vi "Writing direction.vi"(0 "PDF Report IN":refnum<class "PDF Report Class.lvclass">, 2 "Text type":T1, 5 "Phrase refnum":refnum<k24>, 7 "Paragraph refnum":refnum<k24>, 9 "ChapterAutoNumber":refnum<k24>, 11 "error in (no error)":errorcluster, 12 "Section":refnum<k24>, 13 "Title":string) -> (4 "PDF Report OUT":refnum<class "PDF Report Class.lvclass">, 15 "error out":errorcluster)   [LabVIEW 2020, in "Exaprom PDF.lvlib"]
doc: "Version 2.0\nDeveloped by Jean-Marc Simard\nCopyright © 2013, Exaprom Inc.\nAll rights reserved.\nLicense: BSD\n\nWith iTextSharp 4.1.6 (http://itextsharp.sourceforge.net)\nunder Mozilla Public License Version 1.1\n(http://www.mozilla.org/MPL/MPL-1.1.html)"
uses:
  <userlib>/labview-PDF-writer-master/Exaprom PDF.lvlib
  <userlib>/labview-PDF-writer-master/LV Class/PDF Report Class/PDF Report Class.lvclass
  C:/Program Files (x86)/National Instruments/LabVIEW 2020/user.lib/labview-PDF-writer-master/DLL/itextsharp.dll
  DLL/itextsharp.dll
  <userlib>/labview-PDF-writer-master/Controls/Text Controls/Unicode/Type and run direction.ctl
  <userlib>/labview-PDF-writer-master/LV Class/Fonts Class/Font Class.lvclass
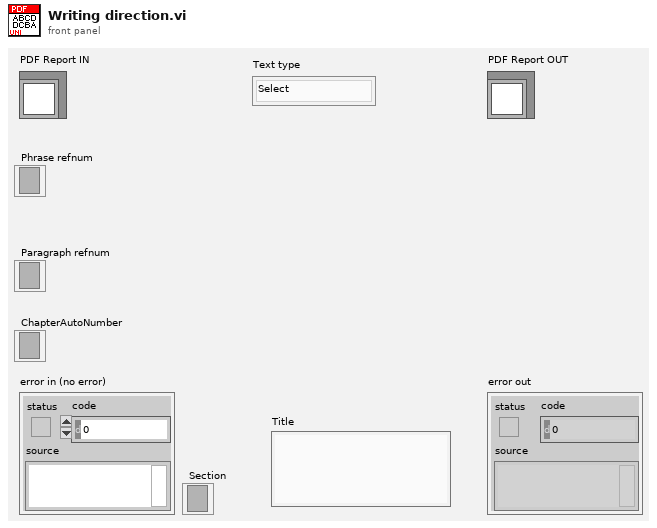
[diagram p1: front panel]
types:
  T1 = typedef "Exaprom PDF.lvlib/Type and run direction.ctl" = enum16{"Select", "ASCII", "UTF-16", "UTF-16 (default)", "UTF-16 (LTR)", "UTF-16 (RTL)"}
  T2 = typedef "Exaprom PDF.lvlib/Font complete cluster.ctl" = cluster{"Name":string, "Size":T3, "Color":T4, "Style":cluster{"Bold":bool, "Italic":bool, "Underline":bool, "Strikeout":bool}, "Type":T5}
  T3 = typedef "Exaprom PDF.lvlib/Font size.ctl" = sgl
  T4 = typedef "Exaprom PDF.lvlib/Font color.ctl" = u32
  T5 = typedef "Exaprom PDF.lvlib/Type and encoding.ctl" = cluster{"Type&direction":T1, "Embedded":bool, "Encoding":string}
  T6 = typedef "Exaprom PDF.lvlib/Page dimensions.ctl" = cluster{"Start at page":i32, "Page Size":T7, "Orientation":T8, "widht":sgl, "height":sgl, "Margin left":sgl, "Margin right":sgl, "Margin top":sgl, "Margin bottom":sgl, "X0":sgl, "X1":sgl, "Y0":sgl, "Y1":sgl}
  T7 = typedef "Exaprom PDF.lvlib/Page size.ctl" = i32
  T8 = typedef "Exaprom PDF.lvlib/Page Orientation.ctl" = enum16{"Portrait", "Landscape"}
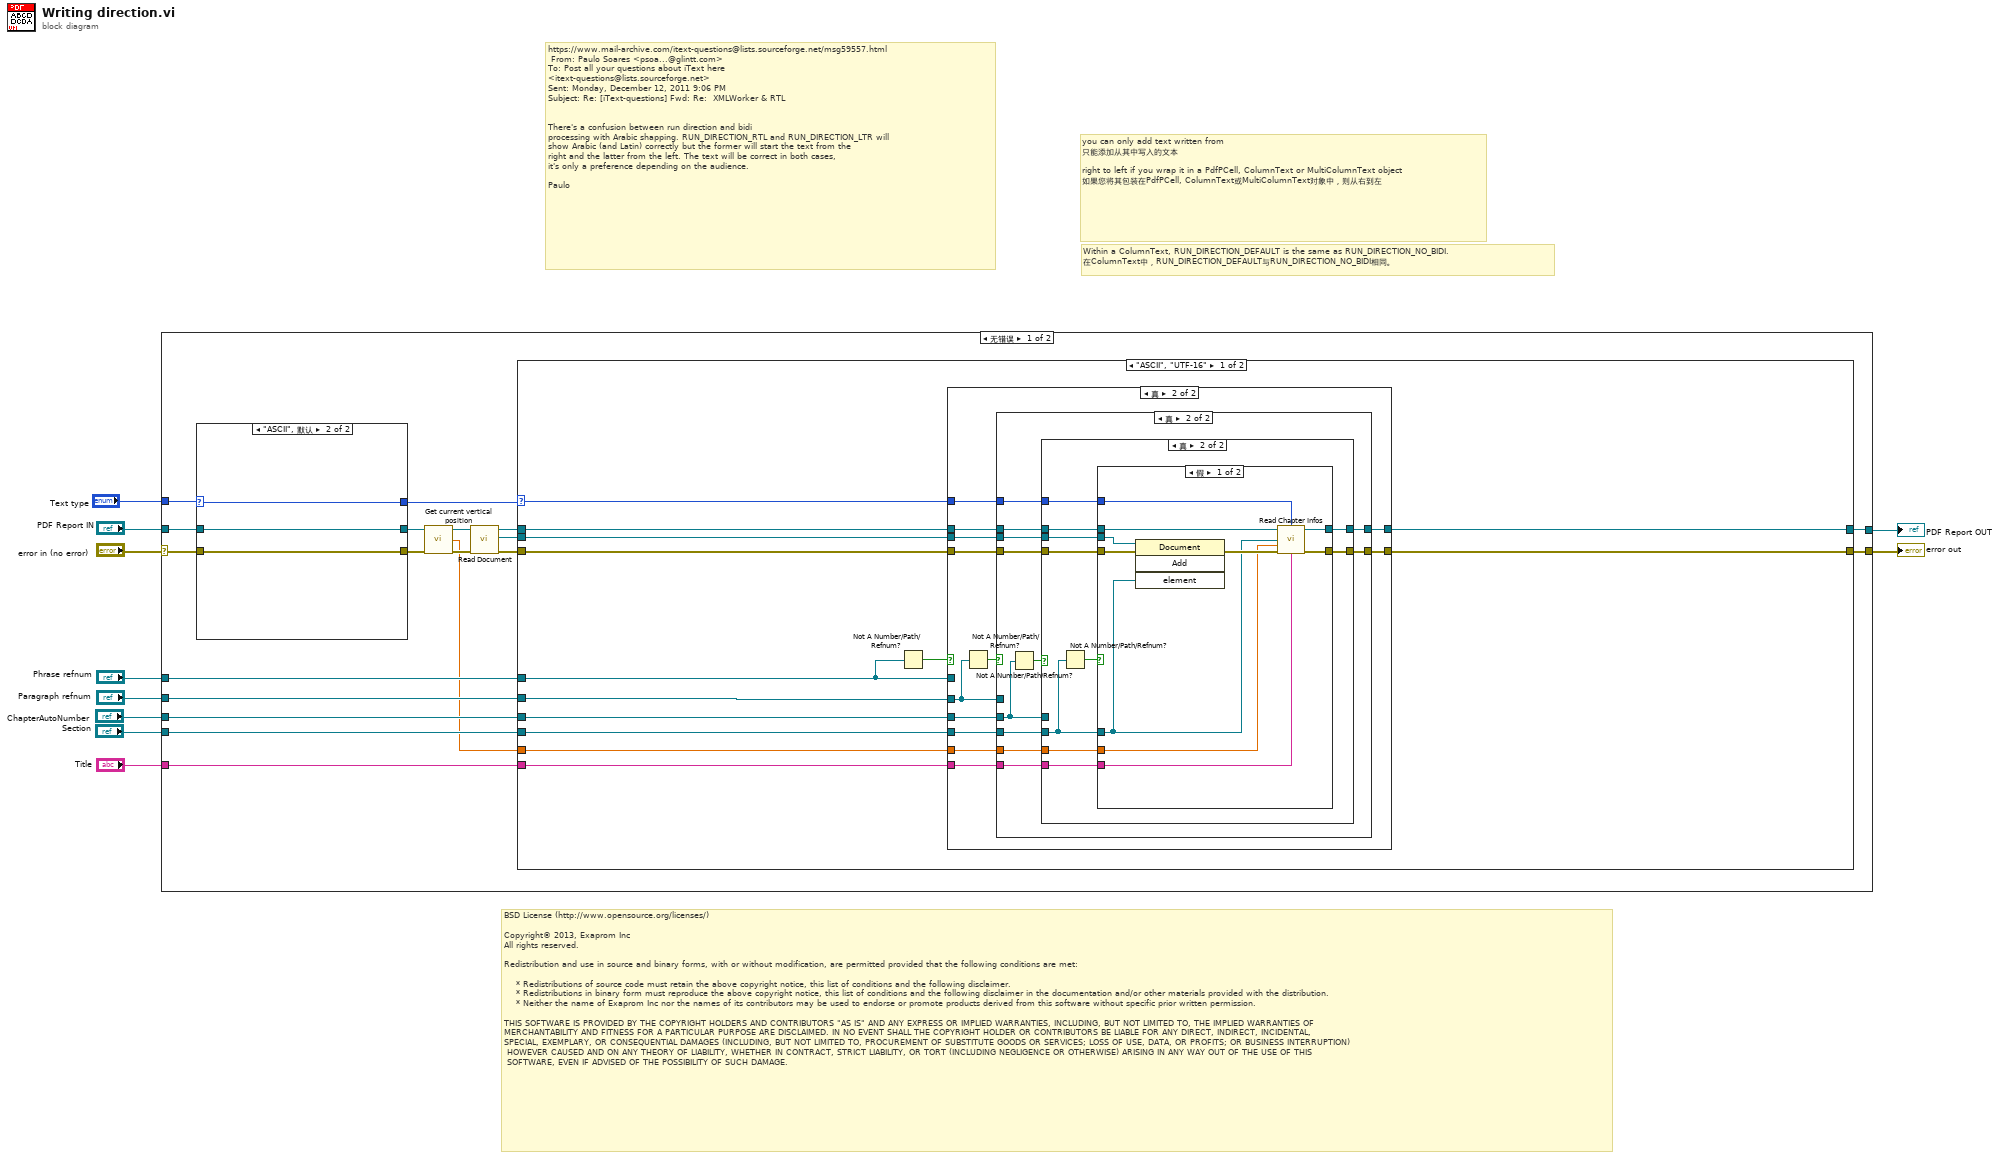
[diagram p0: block diagram]
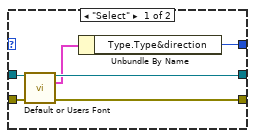
[diagram p2: hidden frame]
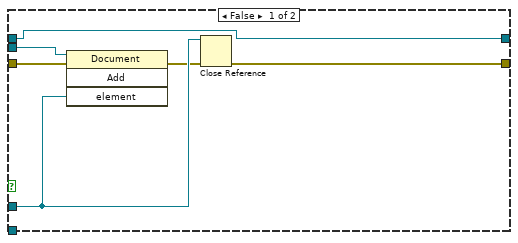
[diagram p3: hidden frame]
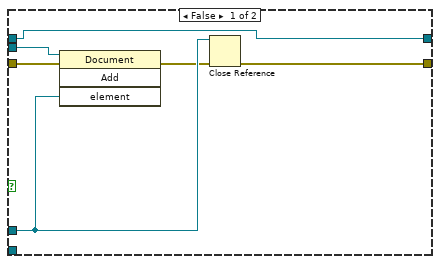
[diagram p4: hidden frame]
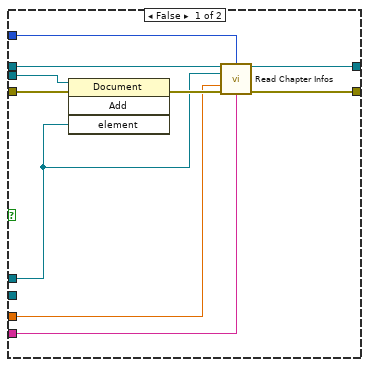
[diagram p5: hidden frame]
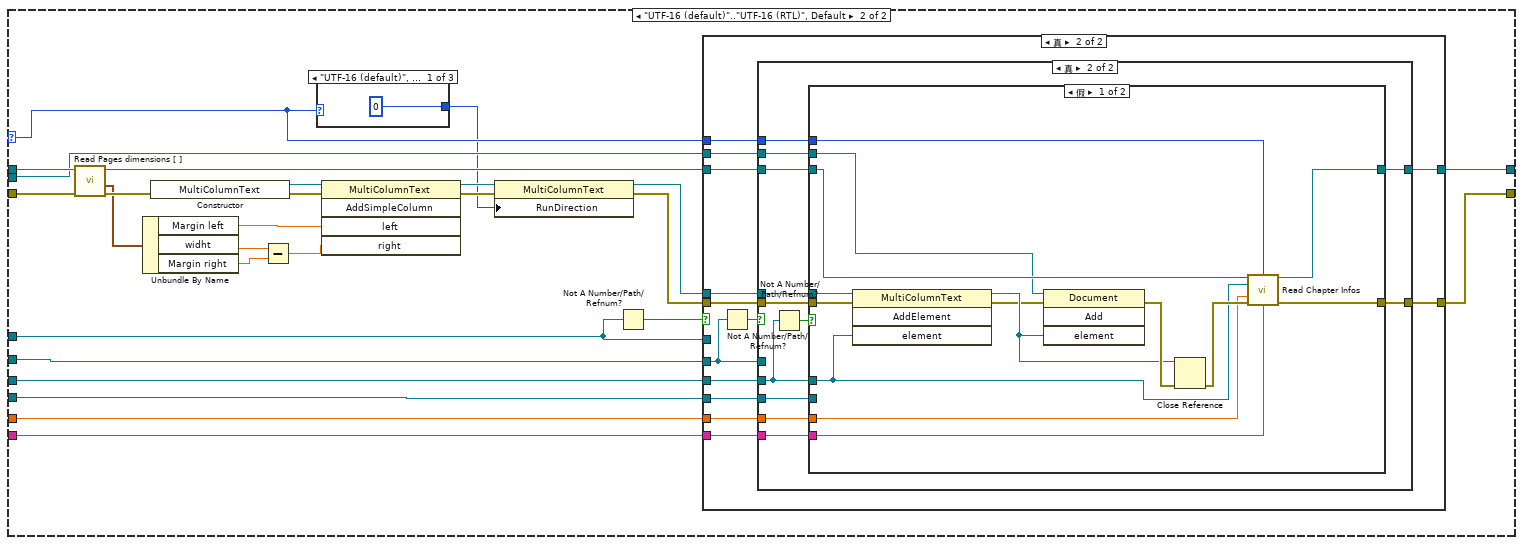
[diagram p7: hidden frame]
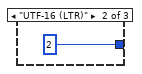
[diagram p8: hidden frame]
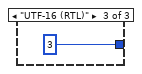
[diagram p9: hidden frame]
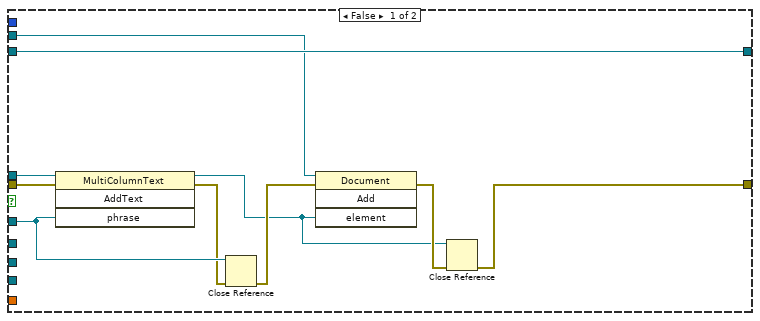
[diagram p10: hidden frame]
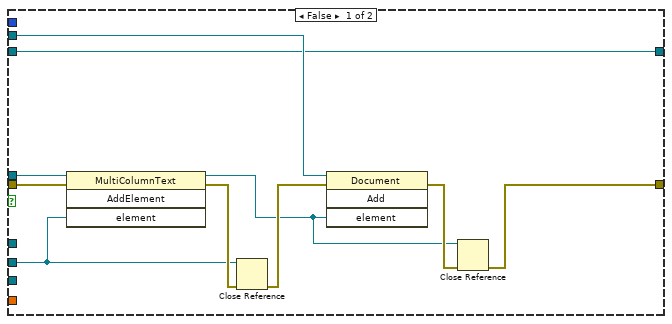
[diagram p11: hidden frame]
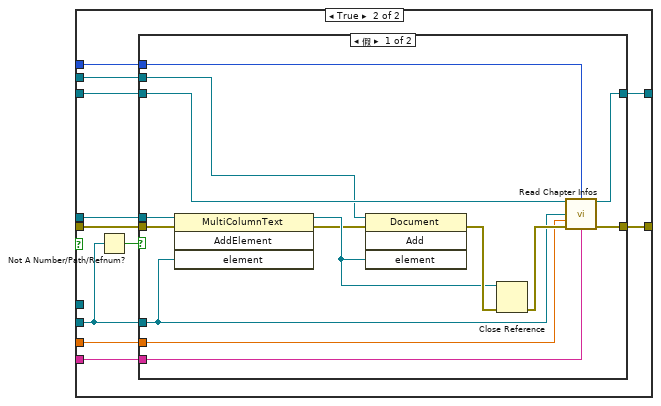
[diagram p12: hidden frame]
diagram:
  # "Within a ColumnText, RUN_DIRECTION_DEFAULT is the same as RUN_DIRECTION_NO_BIDI.\n在ColumnText中，RUN_DIRECTION_DEFAULT与RUN_DIRECTION_NO_BIDI相同。"
  # "you can only add text written from \n只能添加从其中写入的文本\n\nright to left if you wrap it in a PdfPCell, ColumnText or MultiColumnText object\n如果您将其包装在PdfPCell, ColumnText或MultiColumnText对象中，则从右到左"
  # "https://www.mail-archive.com/itext-questions@lists.sourceforge.net/msg59557.html\n From: Paulo Soares <psoa...@glintt.com>\nTo: Post all your questions about iText here \n<itext-questions@lists.sourceforge.net> \nSent: Monday, December 12, 2011 9:06 PM\nSubject: Re: [iText-questions] Fwd: Re:  XMLWorker & RTL\n \n\nThere's a confusion between run direction and bidi \nprocessing with Arabic shapping. RUN_DIRECTION_RTL and RUN_DIRECTION_LTR will \nshow Arabic (and Latin) correctly but the former will start the text from the \nright and the latter from the left. The text will be correct in both cases, \nit's only a preference depending on the audience.\n \nPaulo"
  # "BSD License (http://www.opensource.org/licenses/)\n\nCopyright© 2013, Exaprom Inc\nAll rights reserved.\n\nRedistribution and use in source and binary forms, with or without modification, are permitted provided that the following conditions are met:\n\n    * Redistributions of source code must retain the above copyright notice, this list of conditions and the following disclaimer.\n    * Redistributions in binary form must reproduce the above copyright notice, this list of conditions and the following disclaimer in the documentation and/or other materials provided with the distribution.\n    * Neither the name of Exaprom Inc nor the names of its contributors may be used to endorse or promote products derived from this software without specific prior written permission.\n\nTHIS SOFTWARE IS PROVIDED BY THE COPYRIGHT HOLDERS AND CONTRIBUTORS \"AS IS\" AND ANY EXPRESS OR IMPLIED WARRANTIES, INCLUDING, BUT NOT LIMITED TO, THE IMPLIED WARRANTIES OF \nMERCHANTABILITY AND FITNESS FOR A PARTICULAR PURPOSE ARE DISCLAIMED. IN NO EVENT SHALL THE COPYRIGHT HOLDER OR CONTRIBUTORS BE LIABLE FOR ANY DIRECT, INDIRECT, INCIDENTAL,\nSPECIAL, EXEMPLARY, OR CONSEQUENTIAL DAMAGES (INCLUDING, BUT NOT LIMITED TO, PROCUREMENT OF SUBSTITUTE GOODS OR SERVICES; LOSS OF USE, DATA, OR PROFITS; OR BUSINESS INTERRUPTION)\n HOWEVER CAUSED AND ON ANY THEORY OF LIABILITY, WHETHER IN CONTRACT, STRICT LIABILITY, OR TORT (INCLUDING NEGLIGENCE OR OTHERWISE) ARISING IN ANY WAY OUT OF THE USE OF THIS\n SOFTWARE, EVEN IF ADVISED OF THE POSSIBILITY OF SUCH DAMAGE."
  n1 = case shown="无错误" "error in (no error)" {
    selector: "error in (no error)" -> [w13 w236]
    tunnel: "PDF Report IN" -> [w14 w235]
    tunnel: [w28 w235] -> w9
    tunnel: [w29 w236] -> w8
    tunnel: "Phrase refnum" -> [w27 _]
    tunnel: "Paragraph refnum" -> [w26 _]
    tunnel: "Text type" -> [w16 _]
    tunnel: "ChapterAutoNumber" -> [w22 _]
    tunnel: "Section" -> [w21 _]
    tunnel: "Title" -> [w17 _]
    frame No Error {
      n2 = case shown="\"ASCII\", 默认" w16 {
        selector: w16 -> [_ w38]
        tunnel: [w30 w38] -> w15
        tunnel: w14 -> [w34 w36]
        tunnel: w13 -> [w35 w37]
        tunnel: [w32 w37] -> w12
        tunnel: [w33 w36] -> w11
        frame "Select" {
          n3 = call <userlib>:"Default or Users Font.vi"("PDF Report"=w34, "error in (no error)"=w35) -> ("PDF Report duplicate"=w33:refnum<class "PDF Report Class.lvclass">, "Font OUT"=w31:T2, "error out"=w32:errorcluster)  [unwired: 8 in, 3 out]
          n4 = Unbundle By Name(w31) -> ("Type.Type&direction"=w30:T1)
        }
        frame "ASCII", Default {
        }
      }
      n5 = call <userlib>:"Get current vertical position.vi"("PDF Report In"=w11, "error in (no error)"=w12) -> ("PDF Report duplicate"=w19:refnum<class "PDF Report Class.lvclass">, "GetVerticalPosition (points)"=w18:sgl, "error out"=w20:errorcluster)  [unwired: 11 in]
      n6 = call-dynamic "Read Document.vi"("error in (no error)"=w20, "PDF Report Class in"=w19) -> ("error out"=w25:errorcluster, "Document"=w23:refnum<k24>, "PDF Report Class out"=w24:refnum<class "PDF Report Class.lvclass">)  [unwired: 7 in]
      n7 = case shown="\"ASCII\", \"UTF-16\"" w15 {
        selector: w15 -> [w39 w134]
        tunnel: [w50 w145] -> w29
        tunnel: [w41 w144] -> w28
        tunnel: w27 -> [w47 w143]
        tunnel: w26 -> [w48 w142]
        tunnel: w25 -> [w51 w141]
        tunnel: w24 -> [w43 w140]
        tunnel: w23 -> [w44 w139]
        tunnel: w22 -> [w46 w137]
        tunnel: w21 -> [w45 w138]
        tunnel: w18 -> [w42 w136]
        tunnel: w17 -> [w40 w135]
        frame "ASCII", "UTF-16" {
          n8 = Not A Number/Path/Refnum?(number/path/refnum=w47) -> (NaN/Path/Refnum?=w49:bool)
          n9 = case shown="真" w49 {
            tunnel: [w56 w68] -> w50
            tunnel: w47 -> [w55 _]
            tunnel: w51 -> [w57 w69]
            tunnel: w48 -> [_ w65]
            tunnel: w44 -> [w54 w67]
            tunnel: w46 -> [_ w64]
            tunnel: w45 -> [_ w63]
            tunnel: w43 -> [w52 w62]
            tunnel: w42 -> [_ w61]
            tunnel: [w52 w60] -> w41
            tunnel: w40 -> [_ w59]
            tunnel: w39 -> [_ w58]
            frame False {
              n10 = invoke class="Document" method="Add"(reference=w54, error in=w57, "element"=w55) -> (error out=w53:errorcluster)  [unwired: 1 in, 3 out]
              n11 = Close Reference(reference=w55, error in (no error)=w53) -> (error out=w56:errorcluster)
            }
            frame True {
              n12 = Not A Number/Path/Refnum?(number/path/refnum=w65) -> (NaN/Path/Refnum?=w66:bool)
              n13 = case shown="真" w66 {
                tunnel: w69 -> [w75 w86]
                tunnel: [w74 w85] -> w68
                tunnel: w67 -> [w73 w84]
                tunnel: w65 -> [w72 _]
                tunnel: w64 -> [_ w82]
                tunnel: w63 -> [_ w81]
                tunnel: w62 -> [w70 w80]
                tunnel: w61 -> [_ w79]
                tunnel: [w70 w78] -> w60
                tunnel: w59 -> [_ w77]
                tunnel: w58 -> [_ w76]
                frame False {
                  n14 = invoke class="Document" method="Add"(reference=w73, error in=w75, "element"=w72) -> (error out=w71:errorcluster)  [unwired: 1 in, 3 out]
                  n15 = Close Reference(reference=w72, error in (no error)=w71) -> (error out=w74:errorcluster)
                }
                frame True {
                  n16 = Not A Number/Path/Refnum?(number/path/refnum=w82) -> (NaN/Path/Refnum?=w83:bool)
                  n17 = case shown="真" w83 {
                    tunnel: w86 -> [w96 w106]
                    tunnel: [w94 w105] -> w85
                    tunnel: w84 -> [w95 w104]
                    tunnel: w82 -> [w92 _]
                    tunnel: w81 -> [_ w102]
                    tunnel: w80 -> [w90 w101]
                    tunnel: w79 -> [w91 w100]
                    tunnel: [w89 w99] -> w78
                    tunnel: w77 -> [w88 w98]
                    tunnel: w76 -> [w87 w97]
                    frame False {
                      n18 = invoke class="Document" method="Add"(reference=w95, error in=w96, "element"=w92) -> (error out=w93:errorcluster)  [unwired: 1 in, 3 out]
                      n19 = call <userlib>:"Read Chapter Infos.vi"("PDF Report IN"=w90, "Type and run direction"=w87, "Chapter"=w92, "Y before"=w91, "error in (no error)"=w93, "Title"=w88) -> ("PDF Report OUT"=w89:refnum<class "PDF Report Class.lvclass">, "error out"=w94:errorcluster)  [unwired: 8 in]
                    }
                    frame True {
                      n20 = Not A Number/Path/Refnum?(number/path/refnum=w102) -> (NaN/Path/Refnum?=w103:bool)
                      n21 = case shown="假" w103 {
                        tunnel: w106 -> [w116 w118]
                        tunnel: [w114 w118] -> w105
                        tunnel: w104 -> [w115 _]
                        tunnel: w102 -> [w112 _]
                        tunnel: w101 -> [w110 w117]
                        tunnel: w100 -> [w111 _]
                        tunnel: [w109 w117] -> w99
                        tunnel: w98 -> [w108 _]
                        tunnel: w97 -> [w107 _]
                        frame False {
                          n22 = invoke class="Document" method="Add"(reference=w115, error in=w116, "element"=w112) -> (error out=w113:errorcluster)  [unwired: 1 in, 3 out]
                          n23 = call <userlib>:"Read Chapter Infos.vi"("PDF Report IN"=w110, "Type and run direction"=w107, "Section"=w112, "Y before"=w111, "error in (no error)"=w113, "Title"=w108) -> ("PDF Report OUT"=w109:refnum<class "PDF Report Class.lvclass">, "error out"=w114:errorcluster)  [unwired: 8 in]
                        }
                        frame True {
                        }
                      }
                    }
                  }
                }
              }
            }
          }
        }
        frame "UTF-16 (default)".."UTF-16 (RTL)", Default {
          n24 = call-dynamic "Read Pages dimensions [ ].vi"("error in (no error)"=w141, "PDF Report Class in"=w140) -> ("error out"=w130:errorcluster, "Actual Page dimensions"=w129:T6, "PDF Report Class out"=w121:refnum<class "PDF Report Class.lvclass">)  [unwired: 6 in, 1 out]
          n25 = Unbundle By Name(w129) -> ("Margin left"=w128:sgl, "widht"=w127:sgl, "Margin right"=w126:sgl)
          n26 = constructor class="MultiColumnText"(error in=w130) -> (reference out=w133:refnum<k24>, error out=w132:errorcluster)  [unwired: 2 in, 1 out]
          n27 = Subtract(x=w127, y=w126) -> (x-y=w125:sgl)
          n28 = case shown="\"UTF-16 (default)\", 默认" w134 {
            tunnel: [0 ("RunDirection") 2 ("RunDirection") 3 ("RunDirection")] -> w120
            frame "UTF-16 (default)", Default {
            }
            frame "UTF-16 (LTR)" {
            }
            frame "UTF-16 (RTL)" {
            }
          }
          n29 = invoke class="MultiColumnText" method="AddSimpleColumn"(reference=w133, error in=w132, "left"=w128, "right"=w125) -> (reference out=w124:refnum<k24>, error out=w131:errorcluster)  [unwired: 1 in, 3 out]
          n30 = property class="MultiColumnText"(reference=w124, error in=w131, "RunDirection"=w120) -> (reference out=w119:refnum<k24>, error out=w123:errorcluster)
          n31 = Not A Number/Path/Refnum?(number/path/refnum=w143) -> (NaN/Path/Refnum?=w122:bool)
          n32 = case shown="真" w122 {
            tunnel: [w151 w170] -> w145
            tunnel: w143 -> [w157 _]
            tunnel: w123 -> [w158 w171]
            tunnel: w142 -> [_ w167]
            tunnel: w119 -> [w156 w169]
            tunnel: w137 -> [_ w166]
            tunnel: w138 -> [_ w165]
            tunnel: w136 -> [_ w163]
            tunnel: [w150 w161] -> w144
            tunnel: w121 -> [w150 w162]
            tunnel: w139 -> [w149 w164]
            tunnel: w135 -> [_ w160]
            tunnel: w134 -> [_ w159]
            frame False {
              n33 = invoke class="MultiColumnText" method="AddText"(reference=w156, error in=w158, "phrase"=w157) -> (reference out=w152:refnum<k24>, error out=w155:errorcluster)  [unwired: 1 in, 2 out]
              n34 = Close Reference(reference=w157, error in (no error)=w155) -> (error out=w153:errorcluster)
              n35 = invoke class="Document" method="Add"(reference=w149, error in=w153, "element"=w152) -> (error out=w154:errorcluster)  [unwired: 1 in, 3 out]
              n36 = Close Reference(reference=w152, error in (no error)=w154) -> (error out=w151:errorcluster)
            }
            frame True {
              n37 = Not A Number/Path/Refnum?(number/path/refnum=w167) -> (NaN/Path/Refnum?=w168:bool)
              n38 = case shown="真" w168 {
                tunnel: w171 -> [w177 w193]
                tunnel: [w174 w192] -> w170
                tunnel: w169 -> [w176 w191]
                tunnel: w167 -> [_ _]
                tunnel: w166 -> [w175 w189]
                tunnel: w165 -> [_ w188]
                tunnel: w164 -> [w173 w187]
                tunnel: w163 -> [_ w186]
                tunnel: w162 -> [w172 w185]
                tunnel: [w172 w184] -> w161
                tunnel: w160 -> [_ w183]
                tunnel: w159 -> [_ w182]
                frame False {
                  n39 = invoke class="MultiColumnText" method="AddElement"(reference=w176, error in=w177, "element"=w175) -> (reference out=w178:refnum<k24>, error out=w181:errorcluster)  [unwired: 1 in, 2 out]
                  n40 = Close Reference(reference=w175, error in (no error)=w181) -> (error out=w179:errorcluster)
                  n41 = invoke class="Document" method="Add"(reference=w173, error in=w179, "element"=w178) -> (error out=w180:errorcluster)  [unwired: 1 in, 3 out]
                  n42 = Close Reference(reference=w178, error in (no error)=w180) -> (error out=w174:errorcluster)
                }
                frame True {
                  n43 = Not A Number/Path/Refnum?(number/path/refnum=w189) -> (NaN/Path/Refnum?=w190:bool)
                  n44 = case shown="假" w190 {
                    tunnel: w193 -> [w205 w218]
                    tunnel: [w202 w217] -> w192
                    tunnel: w191 -> [w204 w216]
                    tunnel: w189 -> [w200 _]
                    tunnel: w188 -> [_ w214]
                    tunnel: w187 -> [w196 w211]
                    tunnel: w186 -> [w199 w213]
                    tunnel: w185 -> [w198 w212]
                    tunnel: [w197 w210] -> w184
                    tunnel: w183 -> [w195 w209]
                    tunnel: w182 -> [w194 w208]
                    frame False {
                      n45 = invoke class="MultiColumnText" method="AddElement"(reference=w204, error in=w205, "element"=w200) -> (reference out=w206:refnum<k24>, error out=w203:errorcluster)  [unwired: 1 in, 2 out]
                      n46 = invoke class="Document" method="Add"(reference=w196, error in=w203, "element"=w206) -> (error out=w207:errorcluster)  [unwired: 1 in, 3 out]
                      n47 = Close Reference(reference=w206, error in (no error)=w207) -> (error out=w201:errorcluster)
                      n48 = call <userlib>:"Read Chapter Infos.vi"("PDF Report IN"=w198, "Type and run direction"=w194, "Chapter"=w200, "Y before"=w199, "error in (no error)"=w201, "Title"=w195) -> ("PDF Report OUT"=w197:refnum<class "PDF Report Class.lvclass">, "error out"=w202:errorcluster)  [unwired: 8 in]
                    }
                    frame True {
                      n49 = Not A Number/Path/Refnum?(number/path/refnum=w214) -> (NaN/Path/Refnum?=w215:bool)
                      n50 = case shown="假" w215 {
                        tunnel: w218 -> [w228 w234]
                        tunnel: [w226 w234] -> w217
                        tunnel: w216 -> [w229 _]
                        tunnel: w214 -> [w225 _]
                        tunnel: w213 -> [w224 _]
                        tunnel: w212 -> [w223 w233]
                        tunnel: w211 -> [w222 _]
                        tunnel: [w221 w233] -> w210
                        tunnel: w209 -> [w220 _]
                        tunnel: w208 -> [w219 _]
                        frame False {
                          n51 = invoke class="MultiColumnText" method="AddElement"(reference=w229, error in=w228, "element"=w225) -> (reference out=w231:refnum<k24>, error out=w230:errorcluster)  [unwired: 1 in, 2 out]
                          n52 = invoke class="Document" method="Add"(reference=w222, error in=w230, "element"=w231) -> (error out=w232:errorcluster)  [unwired: 1 in, 3 out]
                          n53 = Close Reference(reference=w231, error in (no error)=w232) -> (error out=w227:errorcluster)
                          n54 = call <userlib>:"Read Chapter Infos.vi"("PDF Report IN"=w223, "Type and run direction"=w219, "Section"=w225, "Y before"=w224, "error in (no error)"=w227, "Title"=w220) -> ("PDF Report OUT"=w221:refnum<class "PDF Report Class.lvclass">, "error out"=w226:errorcluster)  [unwired: 8 in]
                        }
                        frame True {
                        }
                      }
                    }
                  }
                }
              }
            }
          }
        }
      }
    }
    frame Error {
    }
  }
  "PDF Report OUT" <- w9
  "error out" <- w8
